vi "Is Error Cluster.vi"(8 "error in (no error)":errorcluster, 11 "variant":variant) -> (0 "error out":errorcluster, 3 "is error cluster?":bool)   [LabVIEW 2018]
doc: "Returns TRUE if the data type stored in <B>variant</B> is an error cluster."
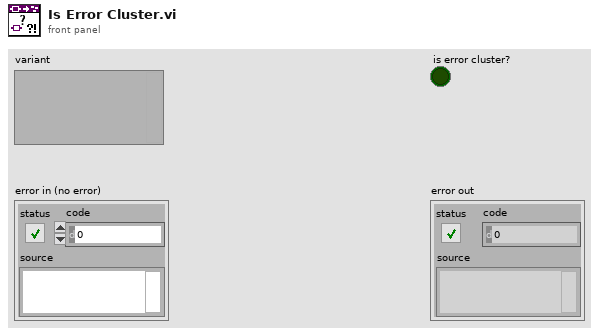
[diagram p1: front panel]
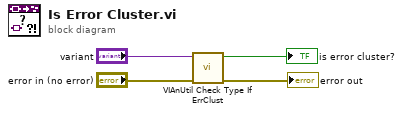
[diagram p0: block diagram]
diagram:
  n1 = call <vilib>:"VIAnUtil Check Type If ErrClust.vi"("error in (no error)"="error in (no error)", "Data In"="variant") -> ("error out"=→"error out":errorcluster, "IsErrClust?"=→"is error cluster?":bool)  [unwired: 8 in]
